vi "Topas4PublicAPIExample.vi"() -> ()   [LabVIEW 2017]
uses:
  E:/UPWORK/Laser Tool/Laser/Topas/Topas4PublicAPI-master/NET_SDK/Topas4Lib.dll
  NET_SDK/Topas4Lib.dll
panel:
  out "Available devices":T1(array[cluster])
  out "Available interactions":string
  in  "Enter serial number of your own device here":string="Orpheus-F-Demo-3981"
  # "If you are seeing lots of erros upon downloading and opening this example, this is LabVIEW configuration problem/pseudo-feature.\nCause and solution is described here http://digital.ni.com/public.nsf/allkb/4742EB60B64BE22186257BCE0053B8FD"
  # "You will notice a lot of \"Property node\" vis have \"Ignore Errors inside node\" set to true.\nIt's so because LabView likes to throw strange errors like \"Error 4: end of file\" for reasons that are unknown to me.\nLikely you'll have to do the same."
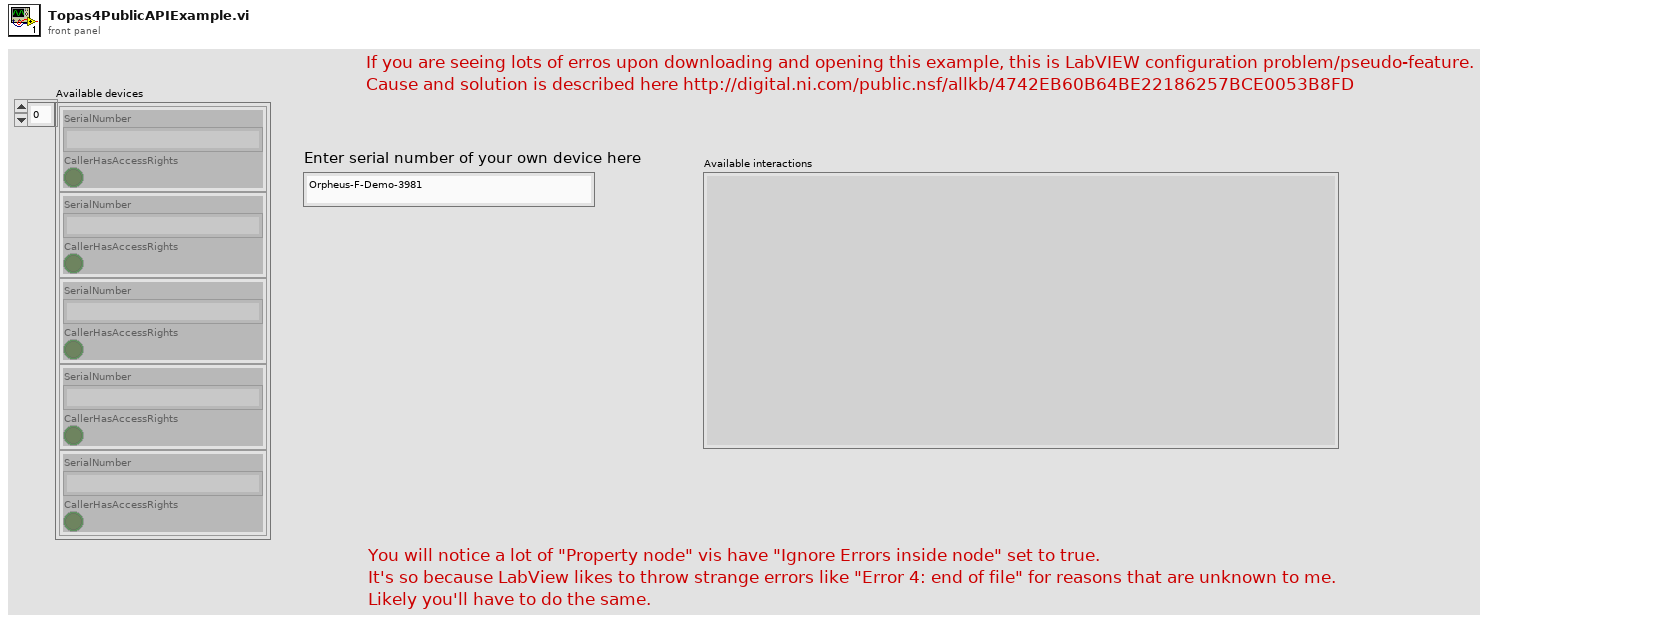
[diagram p1: front panel]
types:
  T1 = cluster{"SerialNumber":string, "CallerHasAccessRights":bool}[]
  T2 = cluster{"SerialNumber":string, "CallerHasAccessRights":bool}
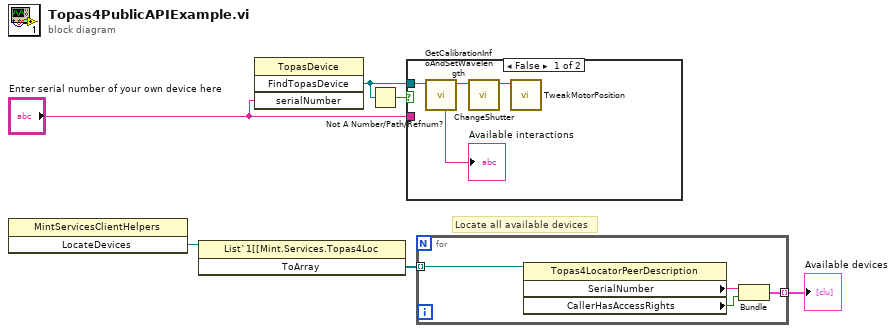
[diagram p0: block diagram]
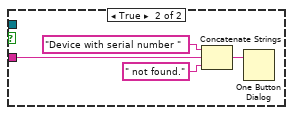
[diagram p2: hidden frame]
diagram:
  # "Locate all available devices"
  n1 = invoke class="MintServicesClientHelpers" method="LocateDevices"() -> ("LocateDevices"=w6:refnum<k24>)  [unwired: 3 in, 2 out]
  n2 = invoke class="List`1[[Mint.Services.Topas4Loc" method="ToArray"(reference=w6) -> ("ToArray"=w5:refnum<k24>[])  [unwired: 2 in, 2 out]
  n3 = invoke class="TopasDevice" method="FindTopasDevice"("serialNumber"="Enter serial number of your own device here") -> ("FindTopasDevice"=w2:refnum<k24>)  [unwired: 3 in, 3 out]
  n4 = Not A Number/Path/Refnum?(number/path/refnum=w2) -> (NaN/Path/Refnum?=w1:bool)
  n5 = case shown="False" w1 {
    tunnel: w2 -> [w8 _]
    tunnel: "Enter serial number of your own device here" -> [_ w13]
    frame False {
      n6 = call "GetCalibrationInfoAndSetWavelength.vi"("Topas In"=w8) -> ("Topas Out"=w7:refnum<k24>, "Available interactions"=→"Available interactions":string)  [unwired: 7 in, 2 out]
      n7 = call "ChangeShutter.vi"("Topas"=w7) -> ("Topas Out"=w9:refnum<k24>)  [unwired: 10 in]
      n8 = call "TweakMotorPosition.vi"("Topas"=w9) -> ()  [unwired: 10 in, 1 out]
    }
    frame True {
      n9 = Concatenate Strings("Device with serial number " ("string"), w13, " not found.") -> (w11:string)
      n10 = One Button Dialog(message=w11) -> ()  [unwired: 1 in, 1 out]
    }
  }
  n11 = for {
    tunnel: w5 -> [w18] mode=indexing
    tunnel: [w15] -> w4 mode=indexing
    n12 = property class="Topas4LocatorPeerDescription"(reference=w18) -> ("SerialNumber"=w17:string, "CallerHasAccessRights"=w16:bool)  [unwired: 1 in, 2 out]
    n13 = Bundle("SerialNumber"=w17, "CallerHasAccessRights"=w16) -> (w15:T2)  [unwired: 1 in]
  }
  "Available devices" <- w4
